vi "Datasheet Generate Table.vi"(0 "ASCII table":string, 1 "Preview?":T1={"Wait? (t)"=TRUE, "ClientPrint? (f)"=FALSE, "Client (\"\")"="", "joinPDF"=FALSE, "Sort Method"=enum."Template", "Export Row (-1=all)"=-1, "Preview"=FALSE, "Estimate Time"=FALSE, "username"="", "jobid"=""}, 2 "Parameters":T3, 3 "Template Record":T5, 5 "error in (no error)":errorcluster, 6 "Paths":T4[](array[typedef]), 7 "Datasheets to Generate":T2[](array[typedef]), 8 "First Item Run":string, 9 "First Item Test Type":string, 10 "First Item Path":string) -> (12 "Paths Out":T4[](array[typedef]), 13 "Datasheets to Generate Out":T2[](array[typedef]), 19 "error out":errorcluster)   [LabVIEW 2011]
uses:
  database/Templates/Template Record.ctl
  Addons/internet/utils/keyedarr.llb/Keyed Array.ctl
  Datasheet Report Info.ctl
  lib/datasheet script data.ctl
  Datasheet Generator Settings.ctl
  Addons/internet/utils/strutil.llb/Case Matching.ctl
panel:
  out "Time":u32
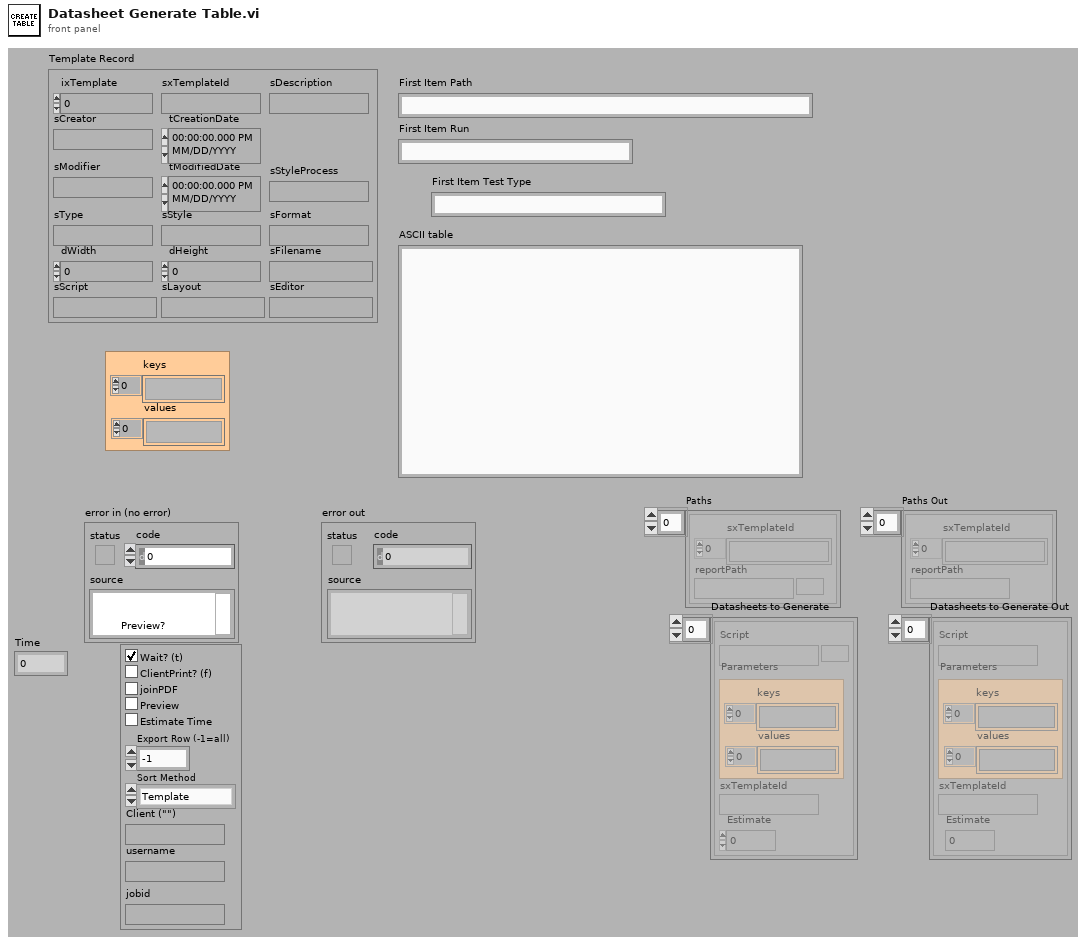
[diagram p1: front panel]
types:
  T1 = typedef "DATASHEET Generator Settings.ctl" = cluster{"Wait? (t)":bool, "ClientPrint? (f)":bool, "Client (\"\")":string, "joinPDF":bool, "Sort Method":enum16{"Item", "Template", "No Sort"}, "Export Row (-1=all)":i32, "Preview":bool, "Estimate Time":bool, "username":string, "jobid":string}
  T2 = typedef "datasheet script data.ctl" = cluster{"Script":path, "Parameters":T3, "sxTemplateId":string, "Estimate":i32}
  T3 = typedef "Keyed Array.ctl" = cluster{"keys":string[], "values":string[]}
  T4 = typedef "Datasheet Report Info.ctl" = cluster{"sxTemplateId":string[], "reportPath":path}
  T5 = typedef "Template Record.ctl" = cluster{"ixTemplate":i32, "sxTemplateId":string, "sDescription":string, "sCreator":string, "tCreationDate":timestamp, "sModifier":string, "tModifiedDate":timestamp, "sType":string, "sStyle":string, "sFormat":string, "dWidth":dbl, "dHeight":dbl, "sFilename":string, "sScript":string, "sLayout":string, "sEditor":string, "sStyleProcess":string}
  T6 = typedef "Case Matching.ctl" = enum16{"a != A", "a == A", "system"}
  T7 = enum16{"open", "replace", "create", "open or create", "replace or create", "replace or create with confirmation"}
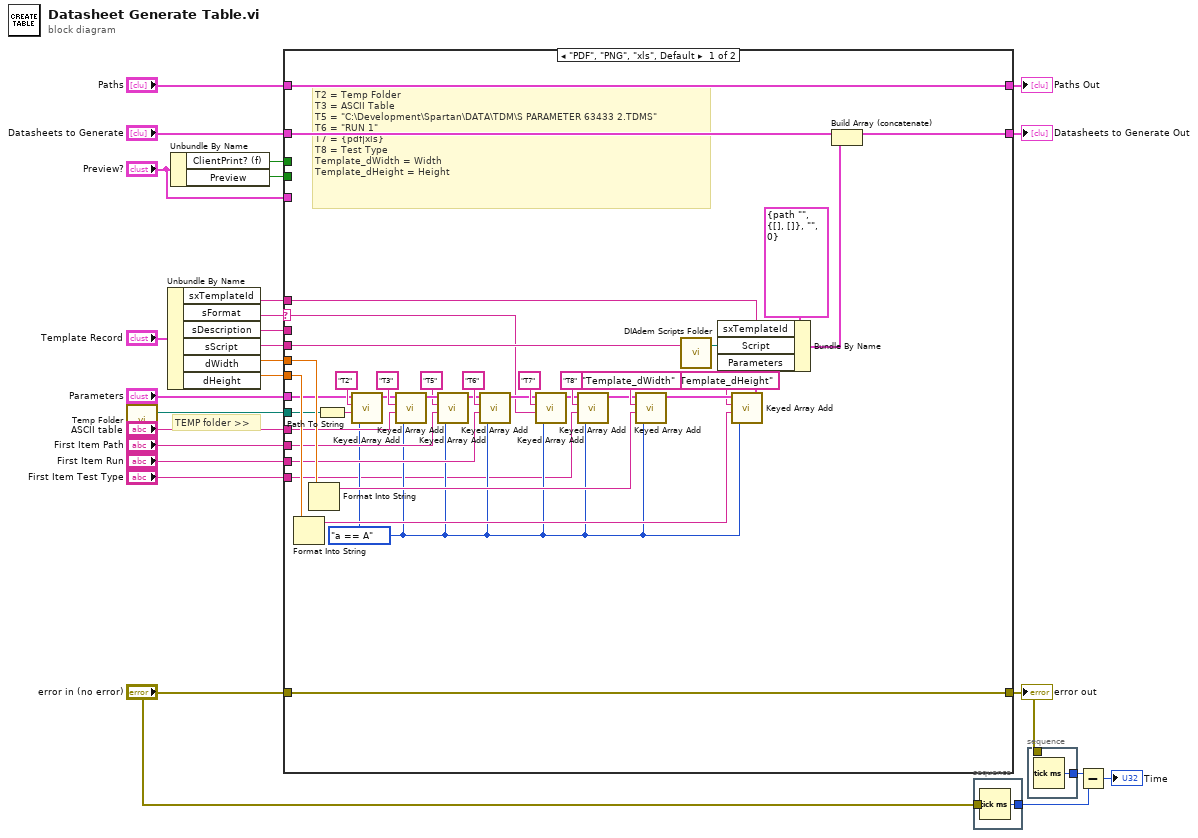
[diagram p0: block diagram]
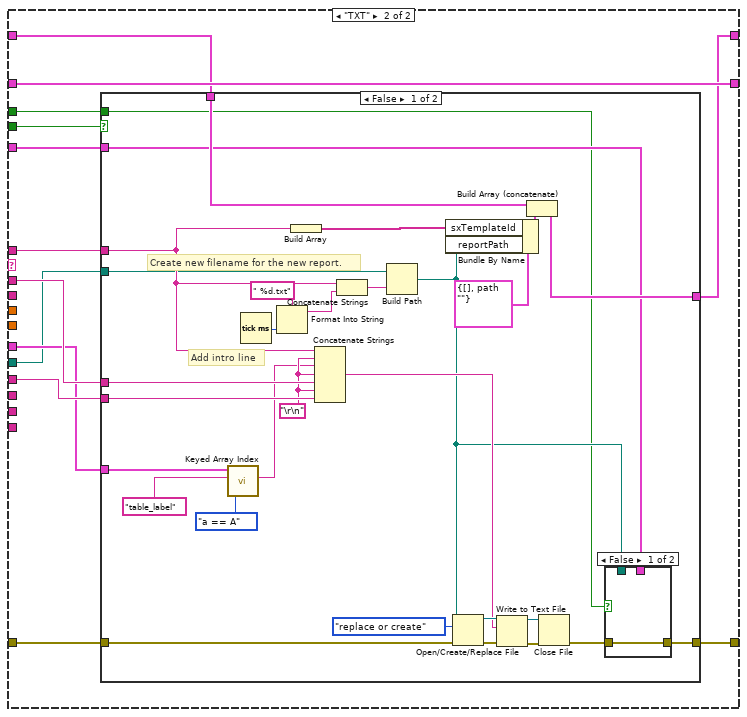
[diagram p2: hidden frame]
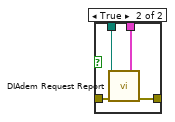
[diagram p3: hidden frame]
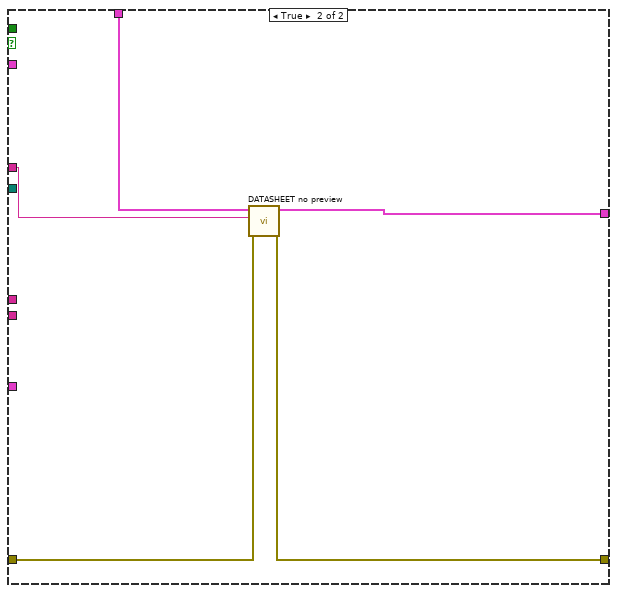
[diagram p4: hidden frame]
diagram:
  # "TEMP folder >>"
  n1 = call "Temp Folder.vi"() -> ("Temp Folder"=w3:path)  [unwired: 3 in]
  n2 = Unbundle By Name("Template Record") -> ("sxTemplateId"=w18:string, "sFormat"=w23:string, "sDescription"=w21:string, "sScript"=w24:string, "dWidth"=w17:dbl, "dHeight"=w16:dbl)
  n3 = Unbundle By Name("Preview?") -> ("ClientPrint? (f)"=w8:bool, "Preview"=w10:bool)
  n4 = case shown="\"PDF\", \"PNG\", \"xls\", Default" w23 {
    selector: w23 -> [w50 _]
    tunnel: [w42 w76] -> w4
    tunnel: "error in (no error)" -> [w42 w75]
    tunnel: w24 -> [w61 _]
    tunnel: "ASCII table" -> [w59 w74]
    tunnel: w21 -> [_ w73]
    tunnel: "First Item Run" -> [w53 _]
    tunnel: "First Item Path" -> [w57 _]
    tunnel: w18 -> [w33 w72]
    tunnel: w17 -> [w63 _]
    tunnel: w16 -> [w62 _]
    tunnel: "Parameters" -> [w40 w71]
    tunnel: "Paths" -> [w37 w69]
    tunnel: [w37 w68] -> w13
    tunnel: "Datasheets to Generate" -> [w36 w70]
    tunnel: [w35 w70] -> w11
    tunnel: w10 -> [_ w67]
    tunnel: "Preview?" -> [_ w66]
    tunnel: w8 -> [_ w65]
    tunnel: w3 -> [w32 w64]
    tunnel: "First Item Test Type" -> [w26 _]
    frame "PDF", "PNG", "xls", Default {
      w27 = Case_Matching."a == A" ("case matching (sensitive)")
      # "T2 = Temp Folder\nT3 = ASCII Table\nT5 = \"C:\\Development\\Spartan\\DATA\\TDM\\S PARAMETER 63433 2.TDMS\"\nT6 = \"RUN 1\"\nT7 = {pdf|xls}\nT8 = Test Type\nTemplate_dWidth = Width\nTemplate_dHeight = Height"
      n5 = Format Into String(w62) -> (resulting string=w46:string)  [unwired: 3 in, 1 out]
      n6 = Format Into String(w63) -> (resulting string=w48:string)  [unwired: 3 in, 1 out]
      n7 = Path To String(path=w32) -> (string=w38:string)
      n8 = call "Keyed Array Add.vi"("case matching (sensitive)"=w27, "value"=w38, "key"="T2" ("format string"), "array in"=w40) -> ("array out"=w39:T3)  [unwired: 3 out]
      n9 = call "Keyed Array Add.vi"("case matching (sensitive)"=w27, "value"=w59, "key"="T3" ("format string"), "array in"=w39) -> ("array out"=w58:T3)  [unwired: 3 out]
      n10 = call "Keyed Array Add.vi"("case matching (sensitive)"=w27, "value"=w57, "key"="T5" ("format string"), "array in"=w58) -> ("array out"=w54:T3)  [unwired: 3 out]
      n11 = call "Keyed Array Add.vi"("case matching (sensitive)"=w27, "value"=w53, "key"="T6" ("format string"), "array in"=w54) -> ("array out"=w51:T3)  [unwired: 3 out]
      n12 = call "Keyed Array Add.vi"("case matching (sensitive)"=w27, "value"=w50, "key"="T7" ("format string"), "array in"=w51) -> ("array out"=w29:T3)  [unwired: 3 out]
      n13 = call "Keyed Array Add.vi"("case matching (sensitive)"=w27, "value"=w26, "key"="T8" ("format string"), "array in"=w29) -> ("array out"=w28:T3)  [unwired: 3 out]
      n14 = call "Keyed Array Add.vi"("case matching (sensitive)"=w27, "value"=w48, "key"="Template_dWidth" ("format string"), "array in"=w28) -> ("array out"=w47:T3)  [unwired: 3 out]
      n15 = call "DIAdem Scripts Folder.vi"("Relative Path (\"\" - Folder)"=w61) -> ("Scripts Folder"=w44:path)  [unwired: 2 out]
      n16 = call "Keyed Array Add.vi"("case matching (sensitive)"=w27, "value"=w46, "key"="Template_dHeight" ("format string"), "array in"=w47) -> ("array out"=w43:T3)  [unwired: 3 out]
      n17 = Bundle By Name(cluster=T2 {"Script"=path "", "Parameters"={"keys"=[], "values"=[]}, "sxTemplateId"="", "Estimate"=0} ("Datasheet"), "sxTemplateId"=w33, "Script"=w44, "Parameters"=w43) -> (w34:T2)
      n18 = Build Array (concatenate)(w36, w34) -> (w35:T2[])
    }
    frame "TXT" {
      n19 = case shown="False" w67 {
        tunnel: [w81 w113] -> w76
        tunnel: w75 -> [w97 w114]
        tunnel: w74 -> [w95 _]
        tunnel: w73 -> [w94 _]
        tunnel: w72 -> [w84 w112]
        tunnel: w71 -> [w91 _]
        tunnel: w69 -> [w88 w116]
        tunnel: [w87 w115] -> w68
        tunnel: w66 -> [w79 _]
        tunnel: w65 -> [w78 _]
        tunnel: w64 -> [w77 _]
        frame False {
          w93 = "\r\n"
          # "Add intro line"
          # "Create new filename for the new report."
          n20 = call "Keyed Array Index.vi"("case matching (sensitive)"=Case_Matching."a == A", "key"="table_label" ("format string"), "array in"=w91) -> ("value"=w90:string)  [unwired: 1 in, 3 out]
          n21 = Tick Count (ms)() -> (millisecond timer value=w98:u32)
          n22 = Format Into String(format string=" %d.txt", w98) -> (resulting string=w106:string)  [unwired: 2 in, 1 out]
          n23 = Build Array(w84) -> (w83:string[])
          n24 = Concatenate Strings(w84, w93, w90, w93, w94, w93, w95) -> (w96:string)
          n25 = Concatenate Strings(w84, w106) -> (w104:string)
          n26 = Build Path(base path=w77, name or relative path=w104) -> (appended path=w80:path)
          n27 = Bundle By Name(cluster=T4 {"sxTemplateId"=[], "reportPath"=path ""} ("report"), "sxTemplateId"=w83, "reportPath"=w80) -> (w85:T4)
          n28 = Open/Create/Replace File(file path (use dialog)=w80, error in=w97, operation (0:open)=T7."replace or create") -> (refnum out=w102:refnum<file>, error out=w101:errorcluster)  [unwired: 4 out]
          n29 = Write to Text File(file (use dialog)=w102, text=w96, error in=w101) -> (refnum out=w100:refnum<file>, error out=w99:errorcluster)  [unwired: 2 out]
          n30 = Build Array (concatenate)(w88, w85) -> (w87:T4[])
          n31 = Close File(refnum=w100, error in=w99) -> (error out=w82:errorcluster)  [unwired: 1 out]
          n32 = case shown="False" w78 {
            tunnel: w82 -> [w107 w111]
            tunnel: [w107 w110] -> w81
            tunnel: w80 -> [_ w109]
            tunnel: w79 -> [_ w108]
            frame False {
            }
            frame True {
              n33 = call "DIAdem Request Report.vi"("Report Path\n(empty - auto PDF in user's folder)"=w109, "generator settings"=w108, "error in (no error)"=w111) -> ("error out"=w110:errorcluster)  [unwired: 12 out]
            }
          }
        }
        frame True {
          n34 = call "DATASHEET no preview.vi"("error in"=w114, "sxTemplateId"=w112, "Paths"=w116) -> ("error out"=w113:errorcluster, "Array"=w115:T4[])  [unwired: 7 out]
        }
      }
    }
  }
  "error out" <- w4
  "Datasheets to Generate Out" <- w11
  "Paths Out" <- w13
  n35 = stacked-sequence {
    tunnel: [w117] -> w6
    tunnel: "error in (no error)" -> [_]
    frame #0 {
      n36 = Tick Count (ms)() -> (millisecond timer value=w117:u32)
    }
  }
  n37 = stacked-sequence {
    tunnel: [w118] -> w7
    tunnel: w4 -> [_]
    frame #0 {
      n38 = Tick Count (ms)() -> (millisecond timer value=w118:u32)
    }
  }
  n39 = Subtract(x=w7, y=w6) -> (x-y=→"Time":u32)
